vi "IsQueueFilled.vi"(7 "N average":i32=10, 8 "error in (no error)":errorcluster, 11 "Array 2":refnum<queue>[](array[refnum])) -> (0 "error out":errorcluster, 1 "ready for stat ?":bool, 2 "elements":cluster{"Intensity Graph 3":u8[][]}[][](array[cluster]), 3 "sum":i32)   [LabVIEW 2018, in "statistics.lvlib"]
uses:
  statistics.lvlib
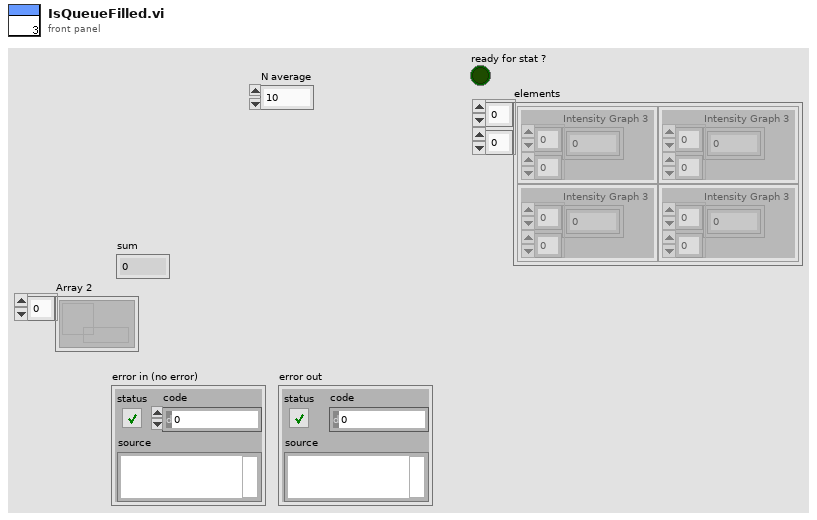
[diagram p1: front panel]
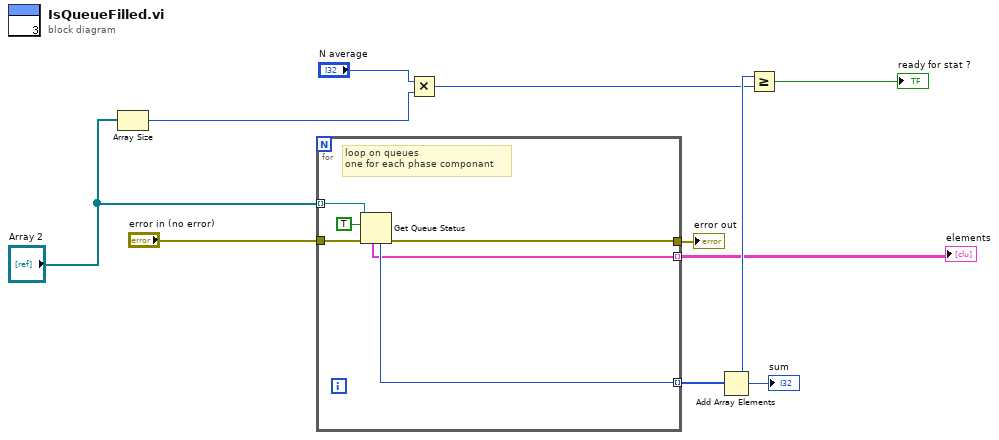
[diagram p0: block diagram]
diagram:
  n1 = Array Size(array="Array 2") -> (size(s)=w9:i32)
  n2 = for {
    tunnel: [w16] -> w4
    tunnel: [w15] -> w10 mode=indexing
    tunnel: "Array 2" -> [w13] mode=indexing
    tunnel: [w11] -> w2 mode=indexing
    tunnel: "error in (no error)" -> [w12]
    # "loop on queues\none for each phase componant"
    n3 = Get Queue Status(queue=w13, return elements? (F)=TRUE, error in (no error)=w12) -> (error out=w16:errorcluster, # elements in queue=w15:i32, elements=w11:cluster{"Intensity Graph":u16[][]}[])  [unwired: 5 out]
  }
  "error out" <- w4
  "elements" <- w2
  n4 = Multiply(x="N average", y=w9) -> (x*y=w6:i32)
  n5 = Add Array Elements(numeric array=w10) -> (sum=w7:i32)
  "sum" <- w7
  n6 = Greater Or Equal?(x=w7, y=w6) -> (x >= y?=→"ready for stat ?":bool)
